vi "Input.vi"(0 "Current * 10^input":dbl, 3 "Sensitivity":dbl, 4 "Scopez":dbl, 5 "Drag":dbl, 6 "FH":dbl, 7 "Signal in":dbl, 8 "FW":dbl, 9 "Scopex":dbl, 10 "Z origin":dbl, 11 "X origin":dbl) -> (1 "Scaled Current":dbl)   [LabVIEW 2017]
uses:
  <userlib>/HapticSTM/Feedbackless - Testdata/Project/feedbackless.lvproj/Proj/Feedbackless Folder/HapticSTM/HapticSTM.lvlib
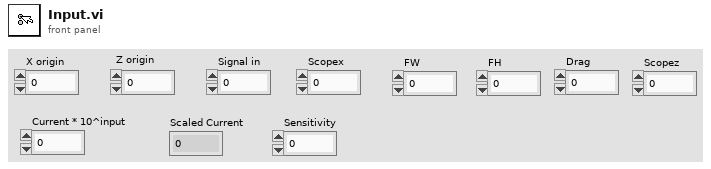
[diagram p1: front panel]
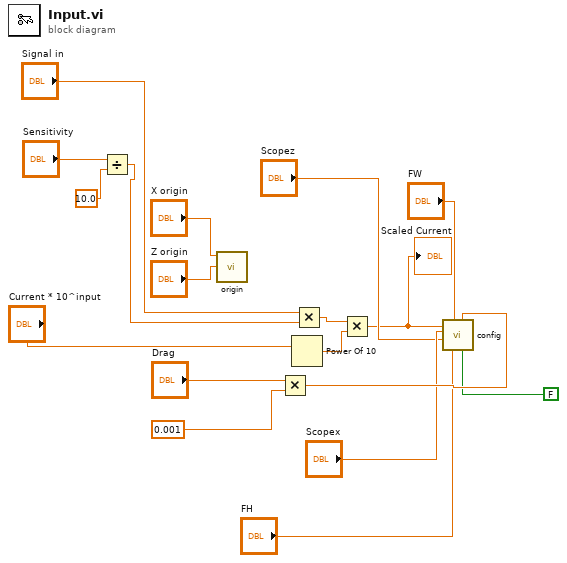
[diagram p0: block diagram]
diagram:
  n1 = Divide(x="Sensitivity", y=10.0) -> (x/y=w3:dbl)
  n2 = call <userlib>:"origin.vi"("zorg"="Z origin", "xorg"="X origin") -> ()  [unwired: 10 in]
  n3 = Multiply(x="Drag", y=0.001) -> (x*y=w14:dbl)
  n4 = Power Of 10(x="Current * 10^input") -> (10^x=w8:dbl)
  n5 = Multiply(x="Signal in", y=w3) -> (x*y=w4:dbl)
  n6 = Multiply(x=w4, y=w8) -> (x*y=w7:dbl)
  "Scaled Current" <- w7
  n7 = call <userlib>:"config.vi"("feedback"=FALSE, "dragc"=w14, "sizeofimgz"="FH", "sizeofimgx"="FW", "scopez"="Scopez", "scopex"="Scopex", "ypos"=w7) -> ()  [unwired: 5 in]
